vi "integration_test.vi"() -> ()   [LabVIEW 2019]
uses:
  <instrlib>/Yokogawa WT200 Series/Yokogawa WT200 Series.lvlib
panel:
  out "Waveform Chart 2":cluster{sgl, sgl, sgl, sgl}(graph)
  out "Waveform Chart":cluster{sgl, sgl, sgl, sgl}(graph)
  out "Integration Values":sgl[](array[numeric]) format="%^.3e"
  out "Measure Values":sgl[](array[numeric]) format="%^.3e"
  in  "Second (0)":u32 max=59 step=1
  in  "error in (no error)":errorcluster
  in  "VISA resource name":refnum<visa-resource-name>
  in  "Minute (0)":u32 max=59 step=1
  in  "Hour (0)":u32 max=10000
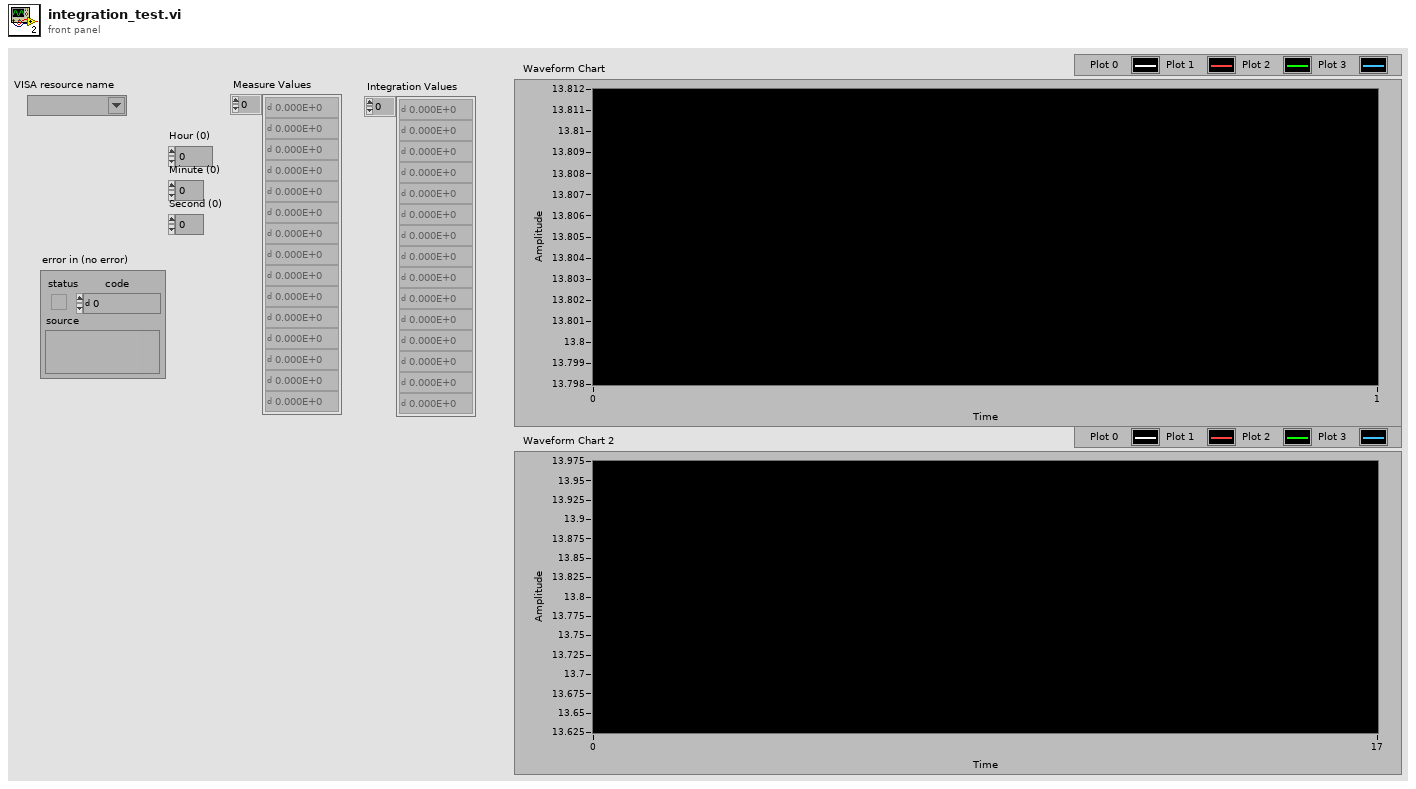
[diagram p1: front panel]
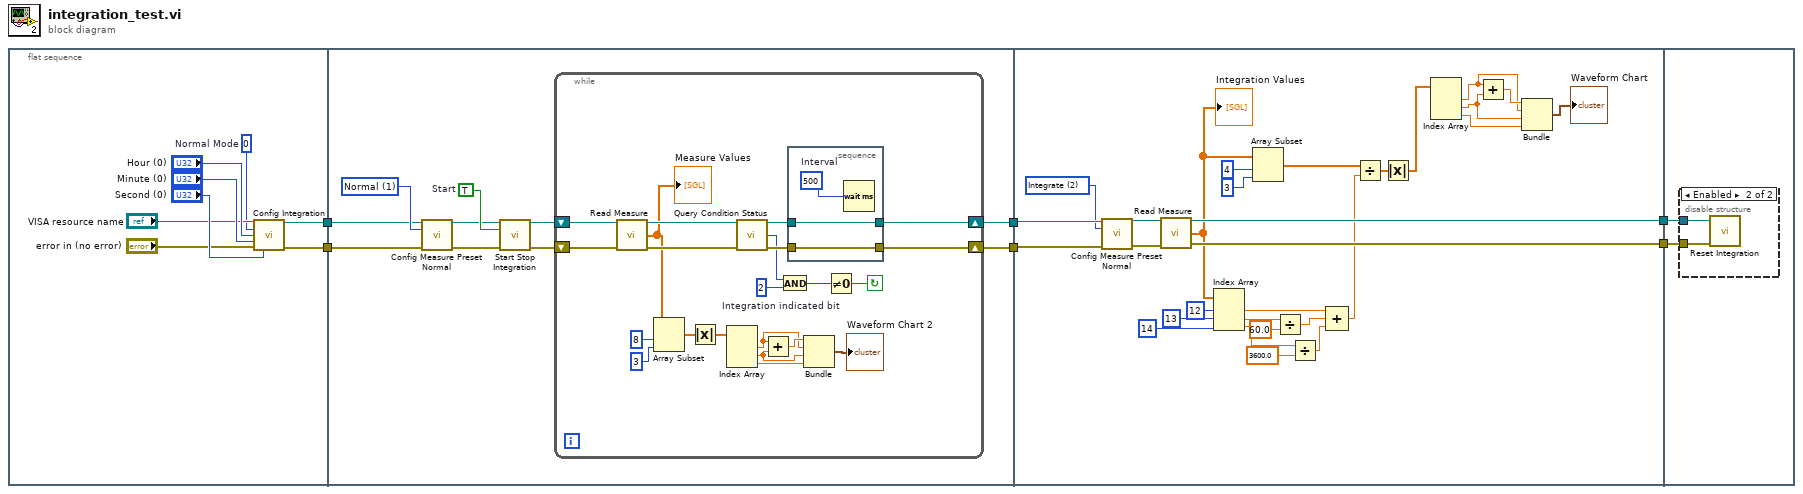
[diagram p0: block diagram]
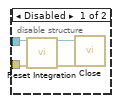
[diagram p2: hidden frame]
diagram:
  n1 = flat-sequence {
    tunnel: [w8] -> w4
    tunnel: [w7] -> w3
    tunnel: [w19] -> w6
    tunnel: [w18] -> w5
    tunnel: w3 -> [w15]
    tunnel: w4 -> [w16]
    tunnel: w6 -> [w78]
    tunnel: w5 -> [w77]
    tunnel: [w73] -> w2
    tunnel: [w72] -> w1
    tunnel: w2 -> [w80]
    tunnel: w1 -> [w79]
    frame #0 {
      w9 = u16 0  # Normal Mode
      n2 = call <instrlib>:"Config Integration.vi"("VISA resource name"="VISA resource name", "Integ Mode (0: Normal)"=w9, "Hour (0)"="Hour (0)", "Minute (0)"="Minute (0)", "error in (no error)"="error in (no error)", "Second (0)"="Second (0)") -> ("VISA resource name out"=w8:refnum<visa-resource-name>, "error out"=w7:errorcluster)  [unwired: 8 in]
    }
    frame #1 {
      w17 = u16 1 items=["Clear", "Normal", "Integrate"] ("Preset Pattern (0: Clear)")
      w22 = TRUE  # Start
      n3 = call <instrlib>:"Config Measure Preset Normal.vi"("VISA resource name"=w16, "Preset Pattern (0: Clear)"=w17, "error in (no error)"=w15) -> ("VISA resource name out"=w21:refnum<visa-resource-name>, "error out"=w20:errorcluster)  [unwired: 11 in]
      n4 = call <instrlib>:"Start Stop Integration.vi"("VISA resource name"=w21, "Start/Stop (F: Stop)"=w22, "error in (no error)"=w20) -> ("VISA resource name out"=w24:refnum<visa-resource-name>, "error out"=w23:errorcluster)  [unwired: 11 in]
      n5 = while {
        shift-left: w24 -> [w38]
        shift-right: [w40] -> w19
        shift-left: w23 -> [w35]
        shift-right: [w42] -> w18
        stop <- w45 continue-if-true
        w46 = u16 2  # Integration indicated bit
        n6 = call <instrlib>:"Read Measure.vi"("VISA resource name"=w38, "error in (no error)"=w35) -> ("VISA resource name out"=w37:refnum<visa-resource-name>, "Measure Value"=w32:sgl[], "error out"=w36:errorcluster)  [unwired: 10 in, 1 out]
        "Measure Values" <- w32
        n7 = Array Subset(array=w32, index=8, length=3) -> (w25:sgl[])
        n8 = Absolute Value(x=w25) -> (abs(x)=w31:sgl[])
        n9 = Index Array(array=w31) -> (element #1=w29:sgl, element #2=w28:sgl, element #3=w27:sgl)  [unwired: 3 in]
        n10 = call <instrlib>:"Query Condition Status.vi"("VISA resource name"=w37, "error in (no error)"=w36) -> ("VISA resource name out"=w41:refnum<visa-resource-name>, "Condition"=w39:u16, "error out"=w43:errorcluster)  [unwired: 11 in]
        n11 = Add(x=w29, y=w28) -> (x+y=w30:sgl)
        n12 = And(x=w39, y=w46) -> (x .and. y?=w44:u16)
        n13 = stacked-sequence {
          tunnel: w43 -> [w48]
          tunnel: [w48] -> w42
          tunnel: w41 -> [w47]
          tunnel: [w47] -> w40
          frame #0 {
            w49 = u32 500  # Interval
            n14 = Wait (ms)(milliseconds to wait=w49) -> ()  [unwired: 1 out]
          }
        }
        n15 = Bundle(w30, w29, w28, w27) -> (→"Waveform Chart 2":cluster{sgl, sgl, sgl, sgl})  [unwired: 1 in]
        n16 = Not Equal To 0?(x=w44) -> (x != 0?=w45:bool)
      }
    }
    frame #2 {
      w76 = u16 2 items=["Clear", "Normal", "Integrate"] ("Preset Pattern (0: Clear)")
      n17 = call <instrlib>:"Config Measure Preset Normal.vi"("VISA resource name"=w78, "Preset Pattern (0: Clear)"=w76, "error in (no error)"=w77) -> ("VISA resource name out"=w75:refnum<visa-resource-name>, "error out"=w74:errorcluster)  [unwired: 11 in]
      n18 = call <instrlib>:"Read Measure.vi"("VISA resource name"=w75, "error in (no error)"=w74) -> ("VISA resource name out"=w73:refnum<visa-resource-name>, "Measure Value"=w61:sgl[], "error out"=w72:errorcluster)  [unwired: 10 in, 1 out]
      "Integration Values" <- w61
      n19 = Index Array(array=w61, index #1=12 ("index"), index #2=13 ("index"), index #3=14 ("index")) -> (element #1=w68:sgl, element #2=w66:sgl, element #3=w65:sgl)
      n20 = Array Subset(array=w61, index=4, length=3) -> (w58:sgl[])
      n21 = Divide(x=w66, y=sgl 60.0) -> (x/y=w67:sgl)
      n22 = Divide(x=w65, y=sgl 3600.0) -> (x/y=w62:sgl)
      n23 = Compound Arithmetic op=ADD(w68, w67, w62) -> (w57:sgl)
      n24 = Divide(x=w58, y=w57) -> (x/y=w56:sgl[])
      n25 = Absolute Value(x=w56) -> (abs(x)=w55:sgl[])
      n26 = Index Array(array=w55) -> (element #1=w53:sgl, element #2=w52:sgl, element #3=w51:sgl)  [unwired: 3 in]
      n27 = Add(x=w53, y=w52) -> (x+y=w54:sgl)
      n28 = Bundle(w54, w53, w52, w51) -> (→"Waveform Chart":cluster{sgl, sgl, sgl, sgl})  [unwired: 1 in]
    }
    frame #3 {
      n29 = disable-structure shown="Enabled" {
        disable-tunnel: w80 -> [w82 w86]
        disable-tunnel: w79 -> [w81 w85]
        frame Disabled {
          n30 = call <instrlib>:"Reset Integration.vi"("VISA resource name"=w82, "error in (no error)"=w81) -> ("VISA resource name out"=w84:refnum<visa-resource-name>, "error out"=w83:errorcluster)  [unwired: 12 in]
          n31 = call <instrlib>:"Close.vi"("VISA resource name"=w84, "error in (no error)"=w83) -> ()  [unwired: 13 in, 1 out]
        }
        frame Enabled {
          n32 = call <instrlib>:"Reset Integration.vi"("VISA resource name"=w86, "error in (no error)"=w85) -> ()  [unwired: 12 in, 2 out]
        }
      }
    }
  }
